vi "20211022_HW00.vi"() -> ()   [LabVIEW 2019]
panel:
  out "N3":dbl
  in  "N2":dbl
  in  "N1":dbl
  in  "Operator":enum16{"+", "-", "*", "/"}(ring)
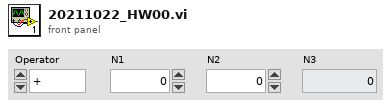
[diagram p1: front panel]
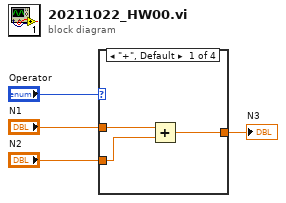
[diagram p0: block diagram]
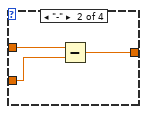
[diagram p2: hidden frame]
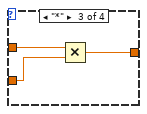
[diagram p3: hidden frame]
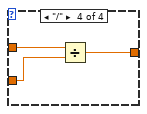
[diagram p4: hidden frame]
diagram:
  n1 = case shown="\"+\", Default" "Operator" {
    tunnel: "N1" -> [w7 w10 w13 w16]
    tunnel: "N2" -> [w6 w9 w12 w15]
    tunnel: [w5 w8 w11 w14] -> w1
    frame "+", Default {
      n2 = Add(x=w7, y=w6) -> (x+y=w5:dbl)
    }
    frame "-" {
      n3 = Subtract(x=w10, y=w9) -> (x-y=w8:dbl)
    }
    frame "*" {
      n4 = Multiply(x=w13, y=w12) -> (x*y=w11:dbl)
    }
    frame "/" {
      n5 = Divide(x=w16, y=w15) -> (x/y=w14:dbl)
    }
  }
  "N3" <- w1
